vi "Get_Driver2.vi"(2 "Driver":string[](array[string]), 8 "error in (no error)":errorcluster caption="错误输入（无错误）", 11 "文件路径 ：":path) -> (0 "error out":errorcluster, 3 "dup path":path)   [LabVIEW 2018]
uses:
  <vilib>/Utility/config.llb/Read Key (String).vi
  <vilib>/Utility/config.llb/NI_LVConfig.lvlib
panel:
  out "Driver":string[](array[string])
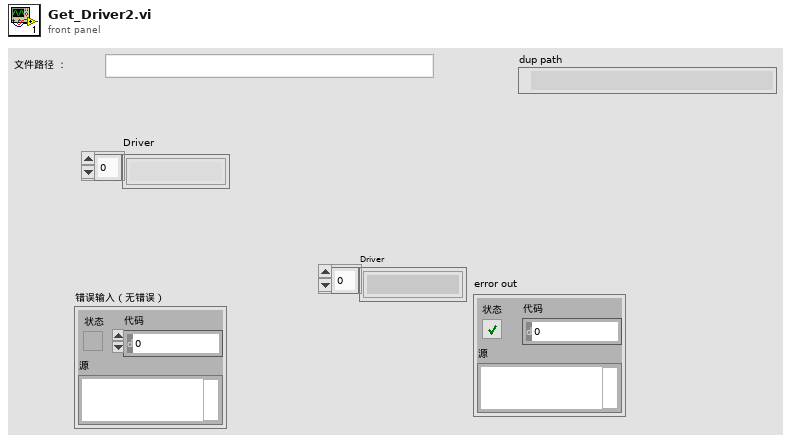
[diagram p1: front panel]
types:
  T1 = enum16{"open", "replace", "create", "open or create", "replace or create", "replace or create with confirmation"}
  T2 = typedef "NI_LVConfig.lvlib/Config Data RefNum.ctl" = refnum<k1>
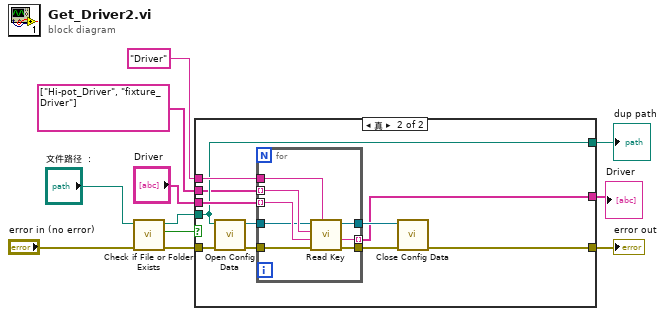
[diagram p0: block diagram]
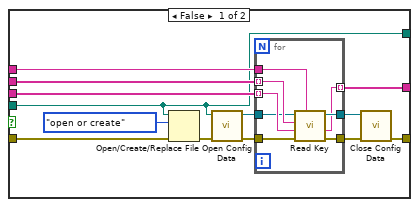
[diagram p2: hidden frame]
diagram:
  n1 = call <vilib>:"Check if File or Folder Exists.vi"("error in (no error)"="error in (no error)", "path"="文件路径 ：") -> ("error out"=w5:errorcluster, "file or folder exists?"=w3:bool, "dup path"=w4:path)  [unwired: 7 in]
  n2 = case shown="真" w3 {
    tunnel: w4 -> [w14 w37]
    tunnel: w5 -> [w16 w43]
    tunnel: "Driver" -> [w15 w42]
    tunnel: [w13 w41] -> w6
    tunnel: "Driver" -> [w20 w40]
    tunnel: [w14 w37] -> w2
    tunnel: string[] ["Hi-pot_Driver", "fixture_Driver"] -> [w19 w35]
    tunnel: [w12 w33] -> w1
    frame False {
      n3 = Open/Create/Replace File(file path (use dialog)=w14, error in=w16, operation (0:open)=T1."open or create" ("操作(0:open)")) -> (error out=w17:errorcluster)  [unwired: 3 in, 2 out]
      n4 = call <vilib>:"Open Config Data.vi"("error in (no error)"=w17, "configuration file path"=w14) -> ("error out"=w18:errorcluster, "refnum"=w21:T2)  [unwired: 7 in, 1 out]
      n5 = for {
        tunnel: w21 -> [w29]
        tunnel: w19 -> [w32] mode=indexing
        tunnel: w15 -> [w28]
        tunnel: w20 -> [w31] mode=indexing
        tunnel: [w30] -> w23
        tunnel: [w27] -> w22
        tunnel: w18 -> [w26]
        tunnel: [w25] -> w12 mode=indexing
        n6 = call-poly <vilib>:"Read Key.vi"("section"=w28, "error in (no error)"=w26, "default value"=w31, "key"=w32, "refnum"=w29) -> ("error out"=w27:errorcluster, "value"=w25:string, "refnum out"=w30:T2)  [unwired: 3 in, 1 out]
      }
      n7 = call <vilib>:"Close Config Data.vi"("error in (no error)"=w22, "refnum"=w23) -> ("error out"=w13:errorcluster)  [unwired: 8 in, 1 out]
    }
    frame True {
      n8 = call <vilib>:"Open Config Data.vi"("error in (no error)"=w43, "configuration file path"=w37) -> ("error out"=w36:errorcluster, "refnum"=w34:T2)  [unwired: 7 in, 1 out]
      n9 = for {
        tunnel: w34 -> [w48]
        tunnel: w35 -> [w51] mode=indexing
        tunnel: w42 -> [w47]
        tunnel: w40 -> [w50] mode=indexing
        tunnel: [w49] -> w39
        tunnel: [w46] -> w38
        tunnel: w36 -> [w45]
        tunnel: [w44] -> w33 mode=indexing
        n10 = call-poly <vilib>:"Read Key.vi"("section"=w47, "error in (no error)"=w45, "default value"=w50, "key"=w51, "refnum"=w48) -> ("error out"=w46:errorcluster, "value"=w44:string, "refnum out"=w49:T2)  [unwired: 3 in, 1 out]
      }
      n11 = call <vilib>:"Close Config Data.vi"("error in (no error)"=w38, "refnum"=w39) -> ("error out"=w41:errorcluster)  [unwired: 8 in, 1 out]
    }
  }
  "error out" <- w6
  "dup path" <- w2
  "Driver" <- w1
